vi "load-leg-zuoqian.vi"(8 "错误输入":errorcluster caption="错误输出") -> (0 "错误输出":errorcluster, 1 "zuoqian3":refnum<vi>, 2 "zuoqian2":refnum<vi>, 3 "zuoqian1":refnum<vi>)   [LabVIEW 2013]
uses:
  <vilib>/picture/3D Picture Control/NI_3D Picture Control.lvlib
panel:
  out "3D Display":refnum<vi>(3d-picture)
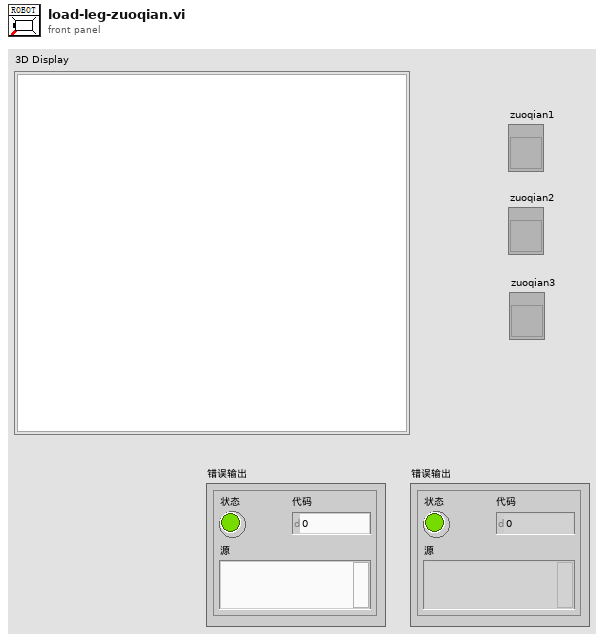
[diagram p1: front panel]
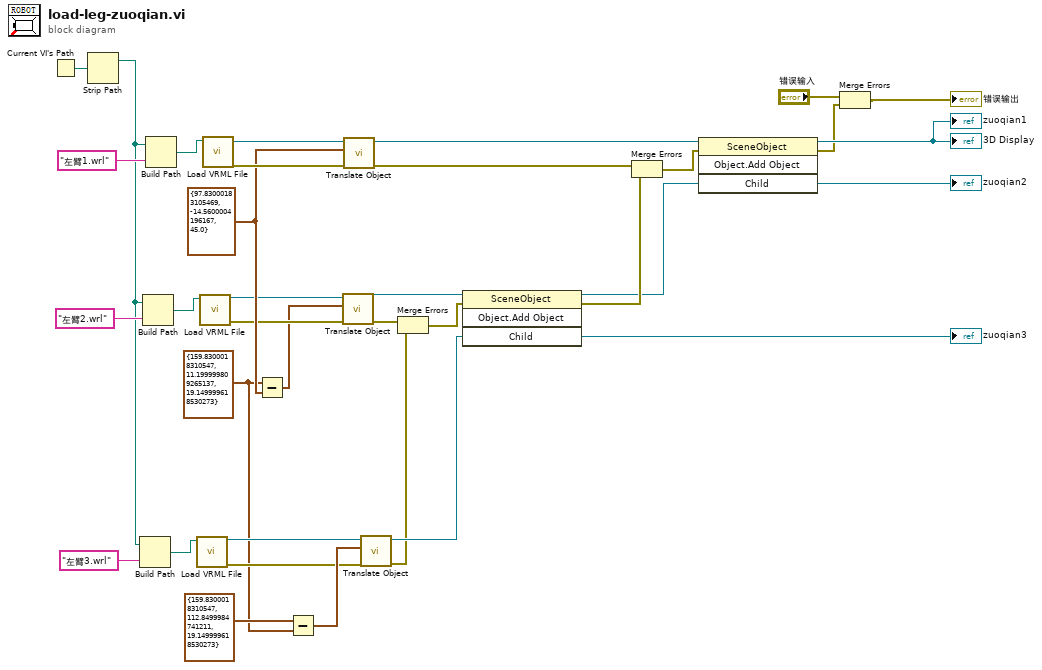
[diagram p0: block diagram]
diagram:
  w6 = cluster{"X":sgl, "Y":sgl, "Z":sgl} {"X"=159.83, "Y"=11.2, "Z"=19.15} ("Translation")
  w25 = cluster{"X":sgl, "Y":sgl, "Z":sgl} {"X"=97.83, "Y"=-14.56, "Z"=45.0} ("Translation")
  n1 = Current VI's Path() -> (path=w35:path)
  n2 = Strip Path(path=w35) -> (stripped path=w28:path)  [unwired: 1 out]
  n3 = Build Path(base path=w28, name or relative path="左臂3.wrl" ("名称或相对路径")) -> (appended path=w29:path)
  n4 = Build Path(base path=w28, name or relative path="左臂2.wrl" ("名称或相对路径")) -> (appended path=w32:path)
  n5 = Build Path(base path=w28, name or relative path="左臂1.wrl" ("名称或相对路径")) -> (appended path=w33:path)
  n6 = call <vilib>:"Load VRML File.vi"("Path"=w29) -> ("error out"=w18:errorcluster, "Scene:Read Scene File"=w19:refnum<vi>)  [unwired: 9 in]
  n7 = call <vilib>:"Load VRML File.vi"("Path"=w32) -> ("error out"=w23:errorcluster, "Scene:Read Scene File"=w24:refnum<vi>)  [unwired: 9 in]
  n8 = call <vilib>:"Load VRML File.vi"("Path"=w33) -> ("error out"=w26:errorcluster, "Scene:Read Scene File"=w27:refnum<vi>)  [unwired: 9 in]
  n9 = Subtract(x=w6, y=w25) -> (x-y=w21:cluster{"X":sgl, "Y":sgl, "Z":sgl})
  n10 = Subtract(x=cluster{"X":sgl, "Y":sgl, "Z":sgl} {"X"=159.83, "Y"=112.85, "Z"=19.15} ("Translation"), y=w6) -> (x-y=w20:cluster{"X":sgl, "Y":sgl, "Z":sgl})
  n11 = call <vilib>:"Translate Object.vi"("error in (no error)"=w23, "Translation"=w21, "Scene.Object In"=w24) -> ("error out"=w14:errorcluster, "Scene.Object Out"=w17:refnum<vi>)  [unwired: 7 in]
  n12 = call <vilib>:"Translate Object.vi"("error in (no error)"=w26, "Translation"=w25, "Scene.Object In"=w27) -> ("error out"=w11:errorcluster, "Scene.Object Out"=w15:refnum<vi>)  [unwired: 7 in]
  n13 = call <vilib>:"Translate Object.vi"("error in (no error)"=w18, "Translation"=w20, "Scene.Object In"=w19) -> ("error out"=w13:errorcluster, "Scene.Object Out"=w16:refnum<vi>)  [unwired: 7 in]
  n14 = Merge Errors(w14, w13) -> (w12:errorcluster)
  n15 = invoke class="SceneObject" method="Object.Add Object"(reference=w17, error in=w12, "Child"=w16) -> (reference out=w8:refnum<vi>, error out=w10:errorcluster, "Child"=→"zuoqian3":refnum<vi>)  [unwired: 1 in, 1 out]
  n16 = Merge Errors(w11, w10) -> (w9:errorcluster)
  n17 = invoke class="SceneObject" method="Object.Add Object"(reference=w15, error in=w9, "Child"=w8) -> (reference out=→"3D Display" →"zuoqian1":refnum<vi>, error out=w2:errorcluster, "Child"=→"zuoqian2":refnum<vi>)  [unwired: 1 in, 1 out]
  n18 = Merge Errors("错误输入", w2) -> (→"错误输出":errorcluster)
